vi "EnqueueMainController.vi"(6 "timeout in ms (-1)":i32=-1, 8 "error in (no error)":errorcluster, 9 "Data":variant, 10 "Message":T1=enum."Exit", 11 "MainQueue":refnum<queue>) -> (0 "error out":errorcluster, 1 "timed out?":bool, 3 "MainQueue out":refnum<queue>)   [LabVIEW 2019, in "MainController.lvlib"]
uses:
  MainController.lvlib
  Cluster - MainControllerMessage.ctl
  Enum - MainState.ctl
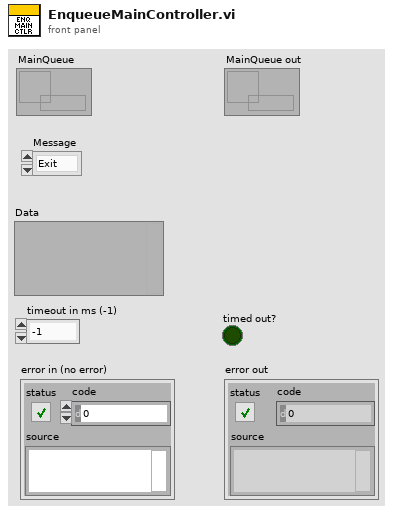
[diagram p1: front panel]
types:
  T1 = typedef "MainController.lvlib/Enum - MainState.ctl" = enum16{"Initialize", "InitUIRefs", "LaunchSettings", "LaunchAutoMode", "LaunchManualMode", "LaunchTestReport", "ConnectHardware", "DisconnectHardware", "HiliteNavItems", "StartAutoMode", "PauseAutoMode", "StopAutoMode", "ShowFlyout", "HideFlyout", "BroadcastSettings", "PickupTestSettings", "BroadcastHW", "AutoTestDone", "DAQStatus", "UpdateCommandBar", "Error", "RecieveError", "Exit"}
  T2 = typedef "MainController.lvlib/Cluster - MainControllerMessage.ctl" = cluster{"Message":T1, "Data":variant}
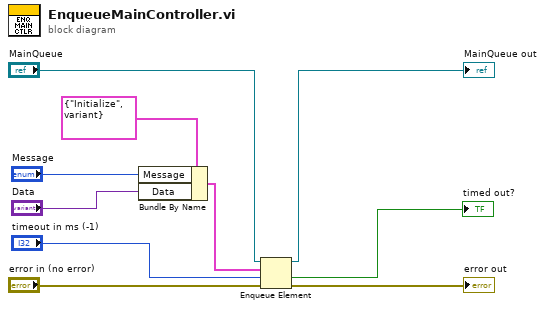
[diagram p0: block diagram]
diagram:
  n1 = Bundle By Name(cluster=T2 {"Message"=enum."Initialize", "Data"=variant} ("Message"), "Message"="Message", "Data"="Data") -> (w4:T2)
  n2 = Enqueue Element(queue="MainQueue", element=w4, timeout in ms (-1)="timeout in ms (-1)", error in (no error)="error in (no error)") -> (queue out=→"MainQueue out":refnum<queue>, timed out?=→"timed out?":bool, error out=→"error out":errorcluster)
